vi "lcd_clear_line (SubVI).vi"(11 "Numeric":dbl) -> ()   [LabVIEW 2015]
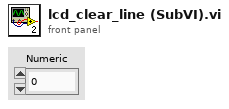
[diagram p1: front panel]
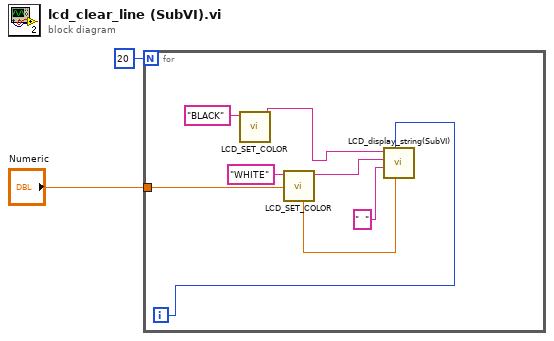
[diagram p0: block diagram]
diagram:
  n1 = for {
    N: 20 -> [_]
    tunnel: "Numeric" -> [w4]
    i -> [w3]
    n2 = call "LCD_SET_COLOR.vi"("String in"="BLACK") -> ("String out"=w9:string)  [unwired: 10 in]
    n3 = call "LCD_SET_COLOR.vi"("String in"="WHITE") -> ("String out"=w7:string)  [unwired: 10 in]
    n4 = call "LCD_display_string(SubVI).vi"("y"=w4, "x"=w3, "String"="  ", "char_color"=w7, "background"=w9) -> ()  [unwired: 7 in]
  }
